vi "CapacitiveTouch_TouchEndEventExe.vi"(8 "error in (no error)":errorcluster, 10 "Event Registration Refnum In":refnum<event-registration>, 11 "Devices In":u64[](array[numeric])) -> (0 "error out":errorcluster, 2 "Event Registration Refnum Out":refnum<event-registration>, 3 "Devices Out":u64[](array[numeric]), 4 "phid":u64, 5 "Event?":bool, 7 "Index":i32)   [LabVIEW 2012, in "Phidget Capacitive Touch.lvlib"]
doc: "${TouchEnd:Header}"
uses:
  <instrlib>/Phidgets/Phidget Capacitive Touch/Phidget Capacitive Touch.lvlib
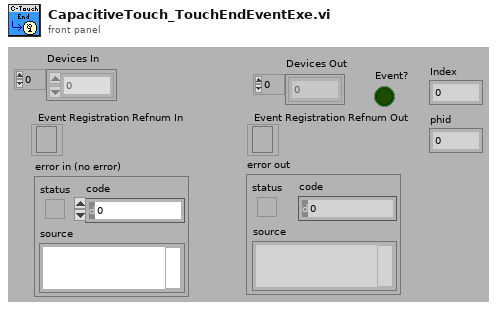
[diagram p1: front panel]
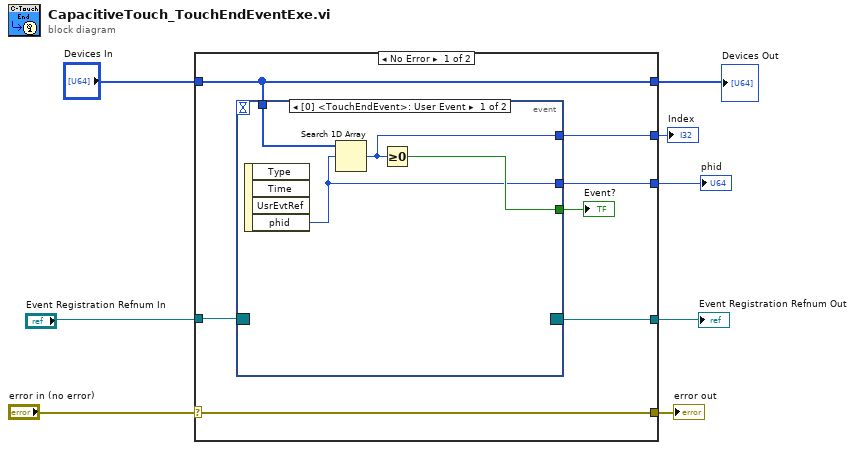
[diagram p0: block diagram]
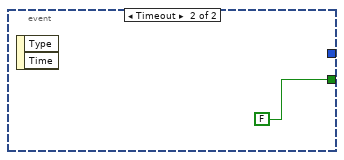
[diagram p2: hidden frame]
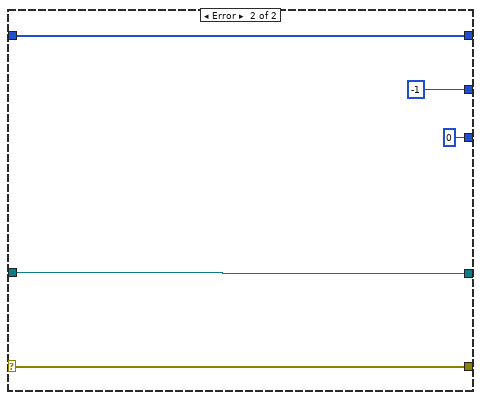
[diagram p3: hidden frame]
diagram:
  n1 = case shown="No Error" "error in (no error)" {
    selector: "error in (no error)" -> [w12 w25]
    tunnel: [w12 w25] -> w7
    tunnel: [w15 w24] -> w1
    tunnel: "Event Registration Refnum In" -> [w14 w24]
    tunnel: [w11 w23] -> w5
    tunnel: "Devices In" -> [w11 w23]
    tunnel: [w10 -1] -> w3
    tunnel: [w9 u64 0 ("phid")] -> w4
    frame No Error {
      n2 = event shown="[0] <TouchEndEvent>: User Event" {
        selector: w14 -> [_ _]
        dyn-events: [_ _] -> w15
        timeout: _ -> [_ _]
        tunnel: [w18 FALSE] -> w13
        tunnel: w11 -> [w19 _]
        tunnel: [w17 _] -> w10
        tunnel: [w16 _] -> w9
        event User Event {
          n3 = event-data() -> ("phid"=w16:u64)  [unwired: 1 in, 3 out]
          n4 = Search 1D Array(1D array=w19, element=w16) -> (index of element=w17:i32)  [unwired: 1 in]
          n5 = Greater Or Equal To 0?(x=w17) -> (x >= 0?=w18:bool)
        }
        event Timeout {
          n6 = event-data() -> ()  [unwired: 1 in, 2 out]
        }
      }
      "Event?" <- w13
    }
    frame Error {
    }
  }
  "error out" <- w7
  "Devices Out" <- w5
  "phid" <- w4
  "Index" <- w3
  "Event Registration Refnum Out" <- w1
